vi "NI VeriStand - Get Channel Value.vi"   [LabVIEW 2020, in "NI_VS Workspace ExecutionAPI.lvlib"]
doc: "Returns values of channels on the target. You can get values for a single channel, multiple channels, or vector values for a single channel. You must manually select the polymorphic instance to use."
uses:
  <vilib>/NI VeriStand/Execution/Workspace/NI_VS Workspace ExecutionAPI.lvlib
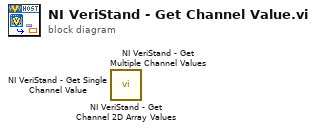
[diagram p0: block diagram]
diagram:
  n1 = call <vilib>:"NI VeriStand - Get Channel 2D Array Values.vi"() -> ()  [unwired: 9 in, 3 out]
  n2 = call <vilib>:"NI VeriStand - Get Multiple Channel Values.vi"() -> ()  [unwired: 9 in, 3 out]
  n3 = call <vilib>:"NI VeriStand - Get Single Channel Value.vi"() -> ()  [unwired: 9 in, 3 out]
